vi "8532_V6.vi"(0 "enum":T11, 7 "set para":T10={"buffer size"=524288, "pci 8532 para"={"Ch"=[1, 1, 1, 1], "inputrange"=[1, 1, 1, 1], "采样频率"=10000, "耦合类型"=1, "预置触发计数器"=1024, "触发模式选择"=0, "ART通道选择"=0, "触发源"=0, "触发方向"=0, "当触发提前时，是否有效"=0, "时钟源"=0, "时钟输入输出源"=0, "是否将时钟信号输入到同步总线"=1}, "segment"={"nReadSizeWords"=8192, "nSegmentCount"=64, "nSegmentSizeWords"=8192}}, 11 "Main Vari in":T1={"Error"={"status"=FALSE, "code"=0, "source"=""}, "Test Info"={"Test Name"="", "Tester"=""}, "StateName"="", "Task Info"={"Accele Task"=[], "Simulate"=FALSE, "采样率"={"AISampleRate"=10123, "CouplingType"=10000, "Butter"=1000}, "Trig"={"PreTrigCNT"=0, "TriggerMode"=enum."中间触发", "TriggerSource"=enum."软件触发", "ATRTriggerChannel"=enum."通道0", "TriggerDir"=enum."下降沿触发", "TrigLevelVolt"=0.0, "bAvailableTrig"=FALSE}, "clock"={"EN"=FALSE, "clocksource"=enum."内部时钟", "outclocksource"=enum."Trig0"}, "delay(S)"=0.0}, "Virb Wave"=[{"t0"=timestamp(3350015091.8292503 s since 1904-01-01), "dt"=0.001, "Y"=array[1000 elements], "attributes"=variant("NI_ChannelName"=variant(string "PXI-6221/ai1"), "NI_UnitDescription"=variant(string "Deg C"))}], "Display Info"=[{"Frequency"=0.0, "RMS"=0.0}, {"Frequency"=0.0, "RMS"=0.0}, {"Frequency"=0.0, "RMS"=0.0}, {"Frequency"=0.0, "RMS"=0.0}, {"Frequency"=0.0, "RMS"=0.0}], "粉尘特性"={"名称"="", "粒径"="", "含水量"=""}, "测试条件"={"初始含氧量"="", "初始压力"="", "测试浓度"="", "点火能量"="", "初始温度"="", "反应器体积[L]"=0.0}, "ch size"=0} {"Task Info"."采样率"."CouplingType" items=["直流耦合", "交流耦合"]}) -> (3 "data?":bool, 6 "wave out":waveform(dbl)[](array[waveform]), 15 "Main Vari out":T1={"Error"={"status"=FALSE, "code"=0, "source"=""}, "Test Info"={"Test Name"="", "Tester"=""}, "StateName"="", "Task Info"={"Accele Task"=[], "Simulate"=FALSE, "采样率"={"AISampleRate"=10123, "CouplingType"=10000, "Butter"=1000}, "Trig"={"PreTrigCNT"=0, "TriggerMode"=enum."中间触发", "TriggerSource"=enum."软件触发", "ATRTriggerChannel"=enum."通道0", "TriggerDir"=enum."下降沿触发", "TrigLevelVolt"=0.0, "bAvailableTrig"=FALSE}, "clock"={"EN"=FALSE, "clocksource"=enum."内部时钟", "outclocksource"=enum."Trig0"}, "delay(S)"=0.0}, "Virb Wave"=[{"t0"=timestamp(3350015091.8292503 s since 1904-01-01), "dt"=0.001, "Y"=array[1000 elements], "attributes"=variant("NI_ChannelName"=variant(string "PXI-6221/ai1"), "NI_UnitDescription"=variant(string "Deg C"))}], "Display Info"=[{"Frequency"=0.0, "RMS"=0.0}, {"Frequency"=0.0, "RMS"=0.0}, {"Frequency"=0.0, "RMS"=0.0}, {"Frequency"=0.0, "RMS"=0.0}, {"Frequency"=0.0, "RMS"=0.0}], "粉尘特性"={"名称"="", "粒径"="", "含水量"=""}, "测试条件"={"初始含氧量"="", "初始压力"="", "测试浓度"="", "点火能量"="", "初始温度"="", "反应器体积[L]"=0.0}, "ch size"=0} {"Task Info"."采样率"."CouplingType" items=["直流耦合", "交流耦合"]})   [LabVIEW 2011]
uses:
  DAQ enum.ctl
  Ctrls/Sample Information.ctl
  Ctrls/Trig.ctl
  Ctrls/clock.ctl
  Ctrls/Task Info.ctl
  Ctrls/Main vari.ctl
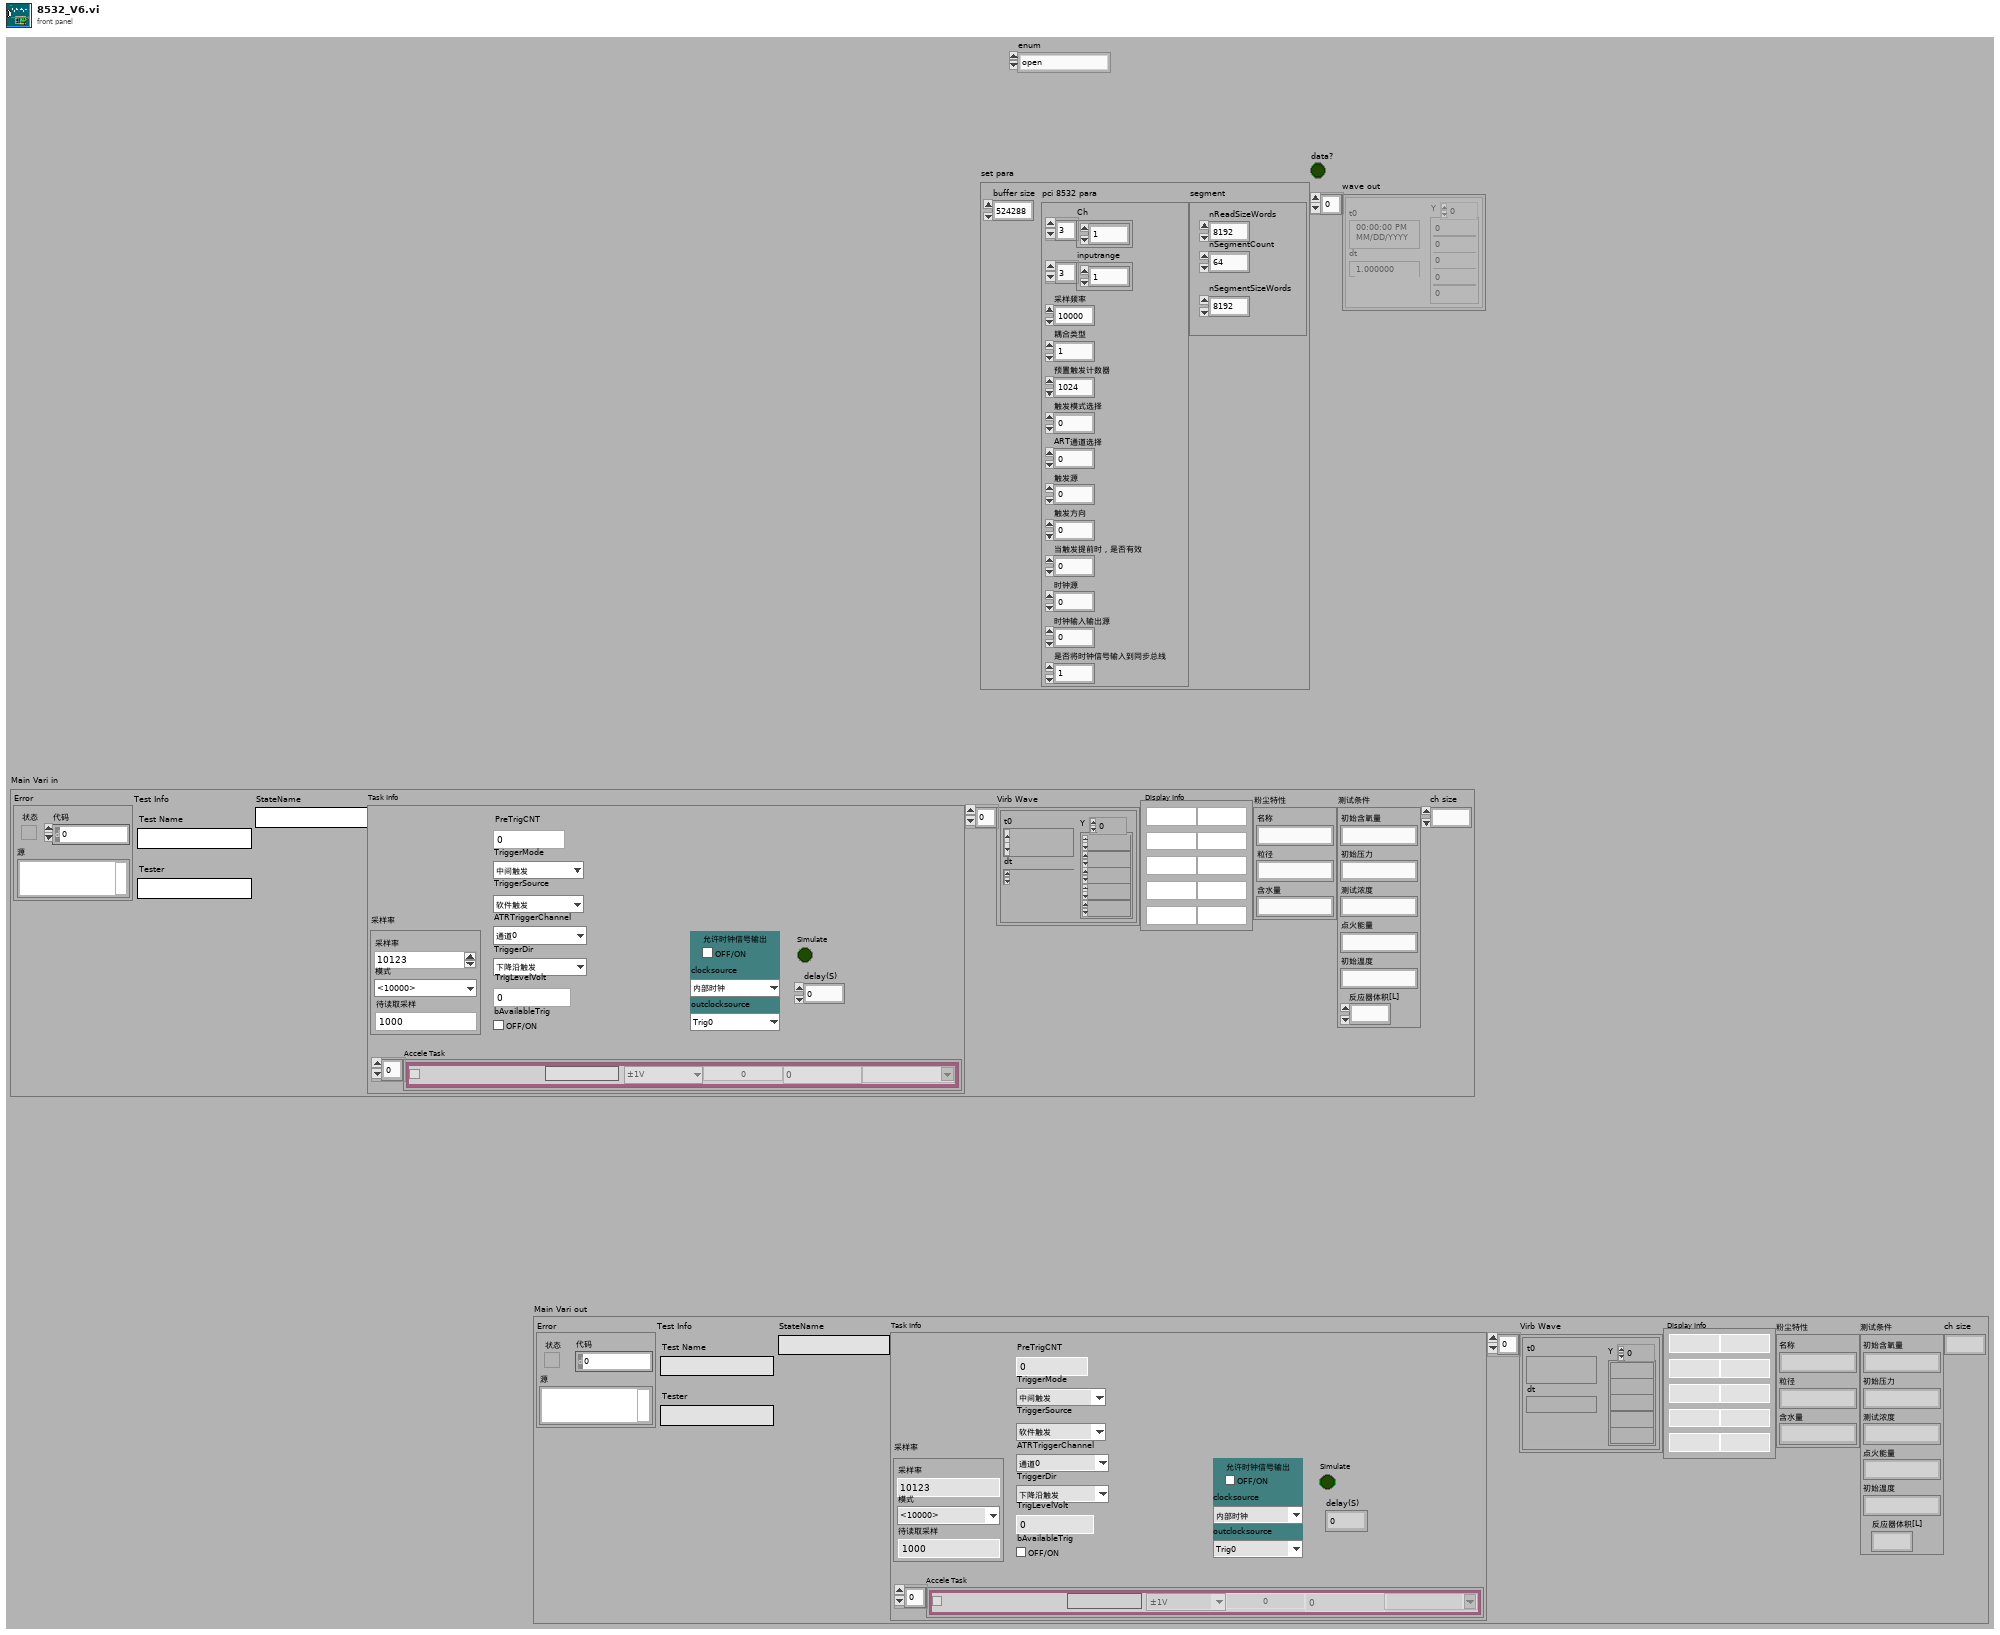
[diagram p1: front panel]
types:
  T1 = typedef "Main vari.ctl" = cluster{"Error":errorcluster, "Test Info":cluster{"Test Name":string, "Tester":string}, "StateName":string, "Task Info":T2, "Virb Wave":waveform(dbl)[], "Display Info":T7, "粉尘特性":T8, "测试条件":T9, "ch size":u8}
  T2 = typedef "Task Info.ctl" = cluster{"Accele Task":T3[], "Simulate":bool, "采样率":T4, "Trig":T5, "clock":T6, "delay(S)":dbl}
  T3 = typedef "Acceleration Channel Config_Ctrls-某型振动实验台测试系统.ctl" = cluster{"Enable":bool, "Name":string, "range":enum16{"±1V", "±5V"}, "SensValue":dbl, "PhysicalName":string, "off":dbl, "Sensunits":string}
  T4 = typedef "Sample Information.ctl" = cluster{"AISampleRate":i32, "CouplingType":i32, "Butter":i32}
  T5 = typedef "Trig.ctl" = cluster{"PreTrigCNT":i32, "TriggerMode":enum16{"中间触发", "后触发", "预触发", "硬件延时触发"}, "TriggerSource":enum16{"软件触发", "DTR信号源", "ATR信号源", "Triger信号触发"}, "ATRTriggerChannel":enum16{"通道0", "通道1", "通道2", "通道3"}, "TriggerDir":enum16{"下降沿触发", "上升沿触发", "上下边没均触发"}, "TrigLevelVolt":sgl, "bAvailableTrig":bool}
  T6 = typedef "clock.ctl" = cluster{"EN":bool, "clocksource":enum16{"内部时钟", "外部时钟"}, "outclocksource":enum16{"Trig0", "Trig1", "Trig2", "Trig3", "Trig4", "Trig5", "Trig6", "Trig7", "PXI_STAR"}}
  T7 = typedef "Display Information_Ctrls-某型振动实验台测试系统.ctl" = cluster{"Frequency":dbl, "RMS":dbl}[]
  T8 = typedef "粉尘特性.ctl" = cluster{"名称":string, "粒径":string, "含水量":string}
  T9 = typedef "测试条件.ctl" = cluster{"初始含氧量":string, "初始压力":string, "测试浓度":string, "点火能量":string, "初始温度":string, "反应器体积[L]":dbl}
  T10 = cluster{"buffer size":i32, "pci 8532 para":cluster{"Ch":i32[], "inputrange":i32[], "采样频率":i32, "耦合类型":i32, "预置触发计数器":i32, "触发模式选择":i32, "ART通道选择":i32, "触发源":i32, "触发方向":i32, "当触发提前时，是否有效":i32, "时钟源":i32, "时钟输入输出源":i32, "是否将时钟信号输入到同步总线":i32}, "segment":cluster{"nReadSizeWords":i32, "nSegmentCount":i32, "nSegmentSizeWords":i32}}
  T11 = typedef "DAQ enum.ctl" = enum16{"open", "config", "start", "read", "stop", "noop", "close"}
  T12 = cluster{"Device":i32, "Event":i32, "state":i32[]}
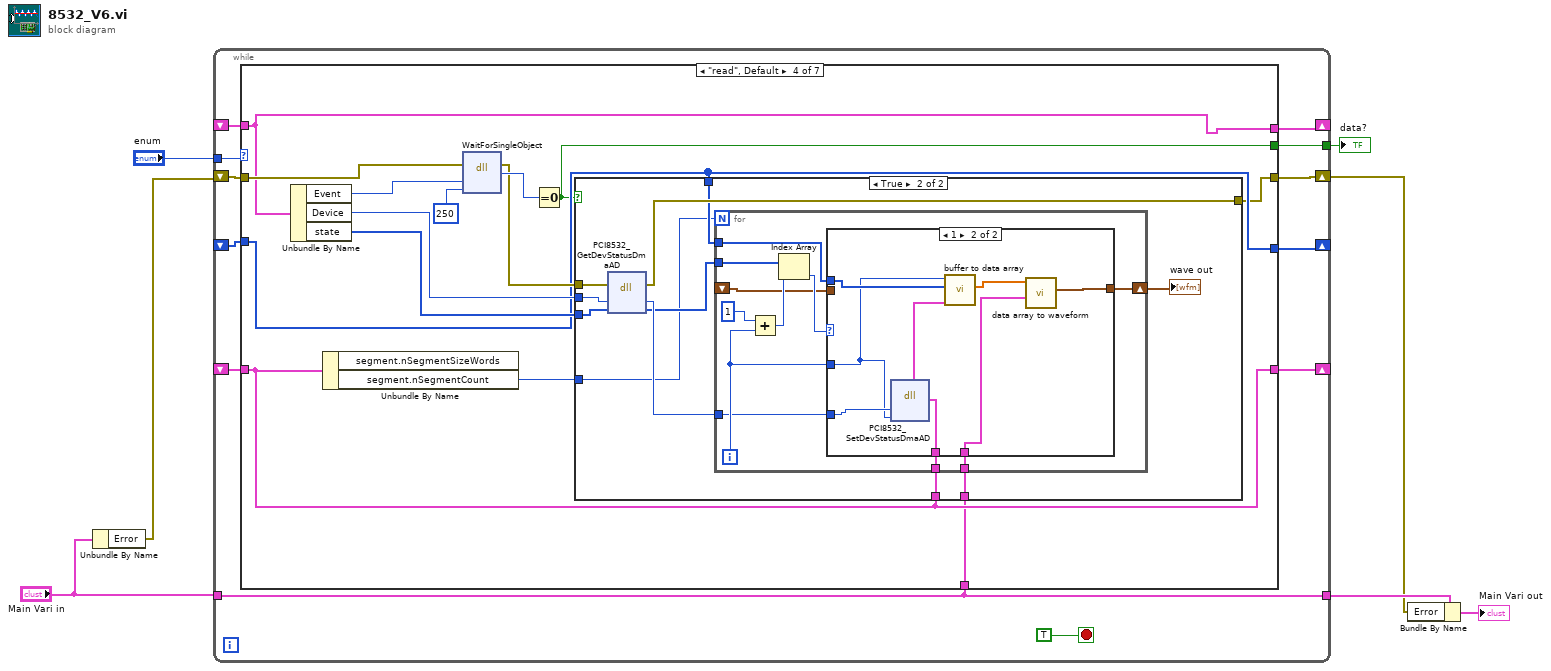
[diagram p0: block diagram]
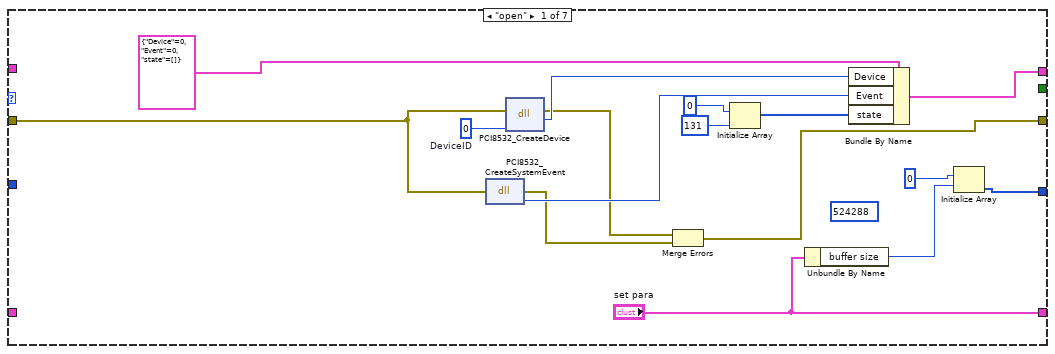
[diagram p2: hidden frame]
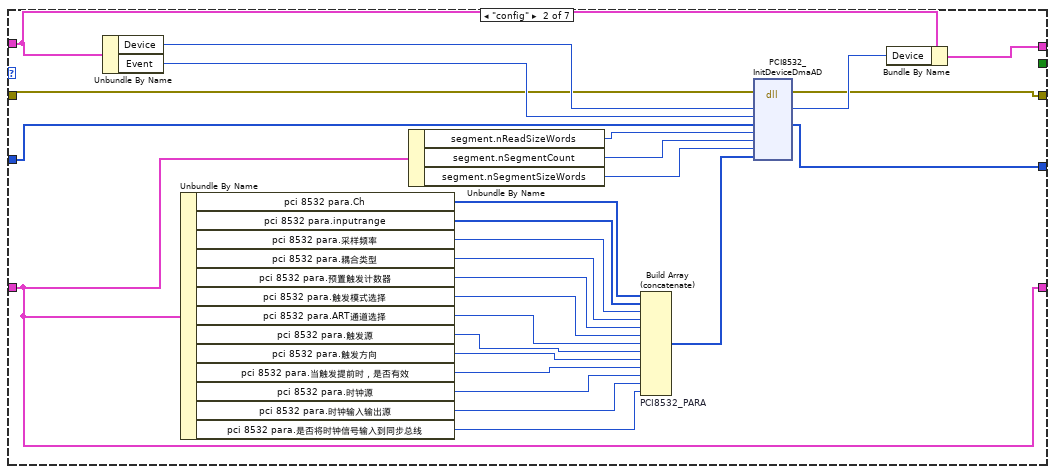
[diagram p3: hidden frame]
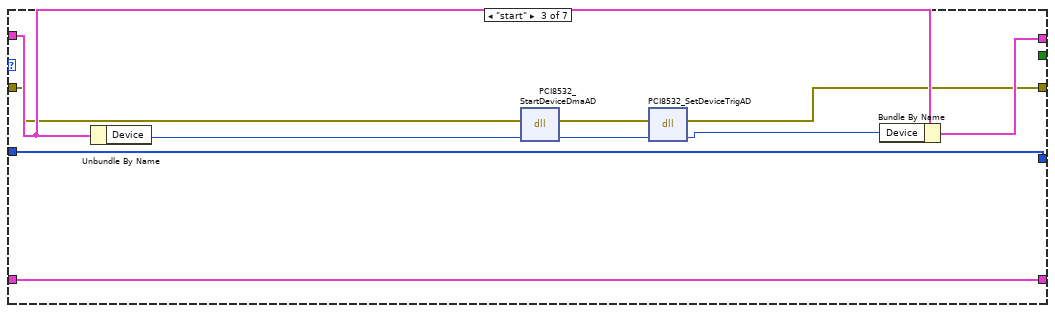
[diagram p4: hidden frame]
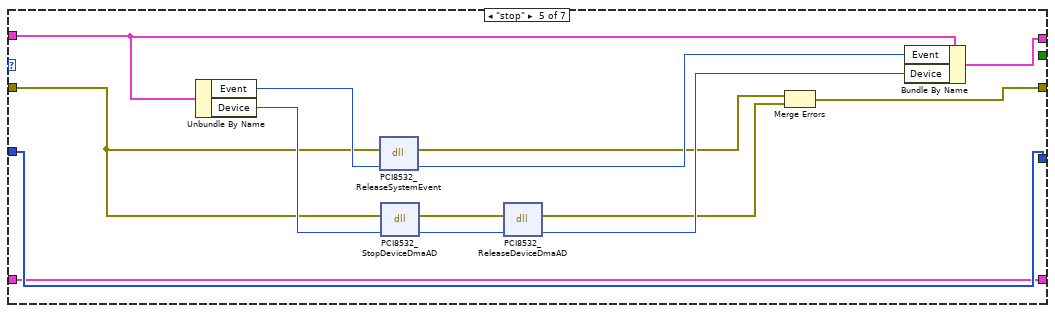
[diagram p7: hidden frame]
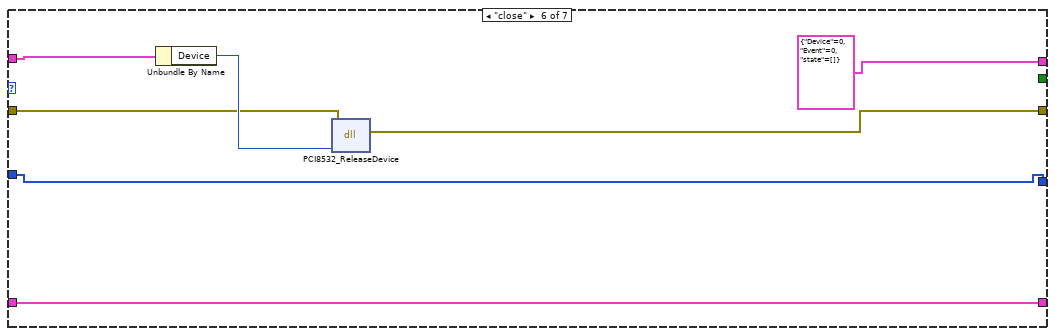
[diagram p8: hidden frame]
diagram:
  n1 = Unbundle By Name("Main Vari in") -> ("Error"=w4:errorcluster)
  n2 = while {
    tunnel: "enum" -> [w18]
    shift-right: [w16] -> _
    shift-left: _ -> [w17]
    shift-right: [w15] -> _
    shift-left: _ -> [w14]
    shift-right: [w12] -> w1
    shift-left: w4 -> [w13]
    shift-right: [w11] -> _
    shift-left: _ -> [w10]
    tunnel: [w9] -> w6
    tunnel: "Main Vari in" -> [w8]
    tunnel: [w8] -> w3
    stop <- TRUE stop-if-true
    n3 = case shown="\"read\", Default" w18 {
      tunnel: w17 -> [_ w58 w68 w78 w129 w138 w142]
      tunnel: [w34 w59 w69 w78 w128 T12 {"Device"=0, "Event"=0, "state"=[]} ("var in") w142] -> w16
      tunnel: [w25 w36 w66 w80 w121 w136 w141] -> w15
      tunnel: w14 -> [_ w56 w66 w80 w121 w136 w141]
      tunnel: w13 -> [w23 w54 w64 w79 w120 w133 w140]
      tunnel: [w22 w55 w65 w77 w119 w134 w140] -> w12
      tunnel: ["set para" w37 w63 w74 w118 w132 w139] -> w11
      tunnel: w10 -> [_ w37 w63 w74 w118 w132 w139]
      tunnel: [_ _ _ w76 _ _ _] -> w9
      tunnel: w8 -> [_ _ _ w73 _ _ _]
      frame "open" {
        (unwired) 524288 ("dimension size")
        w35 = 0  # DeviceID
        n4 = dll-call lib="PCI8532_32" fn="PCI8532_CreateSystemEvent" ("CreateSystemEvent")(error in=w23) -> (error out=w26:errorcluster, "hEvent"=w32:i32)  [unwired: 2 in, 1 out]
        n5 = dll-call lib="PCI8532_32" fn="PCI8532_CreateDevice" label="CreateDevice"(error in=w23, "DeviceID"=w35) -> (error out=w27:errorcluster, w33:i32)  [unwired: 3 in, 1 out]
        n6 = Merge Errors(w27, w26) -> (w22:errorcluster)
        n7 = Initialize Array(0 ("element"), 131 ("dimension size")) -> (w28:i32[])
        n8 = Unbundle By Name("set para") -> ("buffer size"=w20:i32)
        n9 = Bundle By Name(cluster=T12 {"Device"=0, "Event"=0, "state"=[]} ("var in"), "Device"=w33, "Event"=w32, "state"=w28) -> (w34:T12)
        n10 = Initialize Array(u16 0, w20) -> (w25:u16[])
      }
      frame "config" {
        n11 = Unbundle By Name(w58) -> ("Device"=w61:i32, "Event"=w60:i32)
        n12 = Unbundle By Name(w37) -> ("pci 8532 para.Ch"=w50:i32[], "pci 8532 para.inputrange"=w49:i32[], "pci 8532 para.采样频率"=w48:i32, "pci 8532 para.耦合类型"=w47:i32, "pci 8532 para.预置触发计数器"=w46:i32, "pci 8532 para.触发模式选择"=w45:i32, "pci 8532 para.ART通道选择"=w44:i32, "pci 8532 para.触发源"=w43:i32, "pci 8532 para.触发方向"=w42:i32, "pci 8532 para.当触发提前时，是否有效"=w41:i32, "pci 8532 para.时钟源"=w40:i32, "pci 8532 para.时钟输入输出源"=w39:i32, "pci 8532 para.是否将时钟信号输入到同步总线"=w38:i32)
        n13 = Unbundle By Name(w37) -> ("segment.nReadSizeWords"=w53:i32, "segment.nSegmentCount"=w52:i32, "segment.nSegmentSizeWords"=w51:i32)
        n14 = Build Array (concatenate) "PCI8532_PARA"(w50, w49, w48, w47, w46, w45, w44, w43, w42, w41, w40, w39, w38) -> (w62:i32[])
        n15 = dll-call lib="PCI8532_32" fn="PCI8532_InitDeviceDmaAD" label="InitDeviceDmaAD"(error in=w54, "hDevice"=w61, "hDmaEvent"=w60, "ADBuffer"=w56, "nReadSizeWords"=w53, "nSegmentCount"=w52, "nSegmentSizeWords"=w51, "pAPara"=w62) -> (error out=w55:errorcluster, "hDevice"=w57:i32, "ADBuffer"=w36:u16[])  [unwired: 8 in, 1 out]
        n16 = Bundle By Name(cluster=w58, "Device"=w57) -> (w59:T12)
      }
      frame "start" {
        n17 = Unbundle By Name(w68) -> ("Device"=w70:i32)
        n18 = dll-call lib="PCI8532_32" fn="PCI8532_StartDeviceDmaAD" label="StartDeviceDmaAD"(error in=w64, "hDevice"=w70) -> (error out=w71:errorcluster, "hDevice"=w72:i32)  [unwired: 3 in, 1 out]
        n19 = dll-call lib="PCI8532_32" fn="PCI8532_SetDeviceTrigAD" label="SetDeviceTrigAD"(error in=w71, "hDevice"=w72) -> (error out=w65:errorcluster, "hDevice"=w67:i32)  [unwired: 3 in, 1 out]
        n20 = Bundle By Name(cluster=w68, "Device"=w67) -> (w69:T12)
      }
      frame "read", Default {
        n21 = Unbundle By Name(w78) -> ("Event"=w85:i32, "Device"=w82:i32, "state"=w81:i32[])
        n22 = Unbundle By Name(w74) -> ("segment.nSegmentCount"=w75:i32)  [unwired: 1 out]
        n23 = dll-call lib="kernel32" fn="WaitForSingleObject"(error in=w79, "hEvent"=w85, "dwMilliseconds"=250 ("millisecond multiple")) -> (error out=w83:errorcluster, w84:u32)  [unwired: 4 in, 1 out]
        n24 = Equal To 0?(x=w84) -> (x = 0?=w76:bool)
        n25 = case shown="True" w76 {
          tunnel: w83 -> [w87 w98]
          tunnel: [w87 w97] -> w77
          tunnel: w82 -> [_ w96]
          tunnel: w81 -> [_ w95]
          tunnel: w80 -> [_ w93]
          tunnel: w75 -> [_ w91]
          tunnel: w74 -> [_ w90]
          tunnel: w73 -> [_ w88]
          frame False {
          }
          frame True {
            n26 = dll-call lib="PCI8532_32" fn="PCI8532_GetDevStatusDmaAD" ("GetDevStatusDmaAD")(error in=w98, "hDevice"=w96, "pDMAStatus"=w95) -> (error out=w97:errorcluster, "hDevice"=w94:i32, "pDMAStatus"=w92:i32[])  [unwired: 3 in, 1 out]
            n27 = for {
              N: w91 -> [_]
              tunnel: w92 -> [w109]
              tunnel: w93 -> [w107]
              tunnel: w94 -> [w103]
              tunnel: w90 -> [w102]
              shift-right: [w101] -> w89
              shift-left: _ -> [w100]
              tunnel: w88 -> [w99]
              i -> [w105]
              n28 = Add(x=1, y=w105) -> (x+y=w104:i32)
              n29 = Index Array(array=w109, index=w104) -> (element=w108:i32)
              n30 = case shown="1" w108 {
                tunnel: w105 -> [_ w115]
                tunnel: w107 -> [_ w116]
                tunnel: w103 -> [_ w117]
                tunnel: w102 -> [_ w112]
                tunnel: [w110 w114] -> w101
                tunnel: w100 -> [w110 _]
                tunnel: w99 -> [_ w111]
                frame 0, Default {
                }
                frame 1 {
                  n31 = dll-call lib="PCI8532_32" fn="PCI8532_SetDevStatusDmaAD" ("SetDevStatusDmaAD")("hDevice"=w117, "iClrBufferID"=w115) -> ()  [unwired: 6 in, 2 out]
                  n32 = call "buffer to data array.vi"("set para 2"=w112, "buffer"=w116, "i"=w115) -> ("data"=w113:dbl[])  [unwired: 2 in, 6 out]
                  n33 = call "data array to waveform.vi"("Main Vari"=w111, "data"=w113) -> ("wave out"=w114:waveform(dbl)[])  [unwired: 2 in, 7 out]
                }
              }
            }
            "wave out" <- w89
          }
        }
      }
      frame "stop" {
        n34 = Unbundle By Name(w129) -> ("Event"=w130:i32, "Device"=w122:i32)
        n35 = dll-call lib="PCI8532_32" fn="PCI8532_ReleaseSystemEvent" label="ReleaseSystemEvent"(error in=w120, "hEvent"=w130) -> (error out=w125:errorcluster, "hEvent"=w127:i32)  [unwired: 3 in, 1 out]
        n36 = dll-call lib="PCI8532_32" fn="PCI8532_StopDeviceDmaAD" label="StopDeviceDmaAD"(error in=w120, "hDevice"=w122) -> (error out=w123:errorcluster, "hDevice"=w131:i32)  [unwired: 3 in, 1 out]
        n37 = dll-call lib="PCI8532_32" fn="PCI8532_ReleaseDeviceDmaAD" label="ReleaseDeviceDmaAD"(error in=w123, "hDevice"=w131) -> (error out=w124:errorcluster, "hDevice"=w126:i32)  [unwired: 3 in, 1 out]
        n38 = Merge Errors(w125, w124) -> (w119:errorcluster)
        n39 = Bundle By Name(cluster=w129, "Event"=w127, "Device"=w126) -> (w128:T12)
      }
      frame "close" {
        n40 = Unbundle By Name(w138) -> ("Device"=w137:i32)
        n41 = dll-call lib="PCI8532_32" fn="PCI8532_ReleaseDevice" label="ReleaseDevice"(error in=w133, "hDevice"=w137) -> (error out=w134:errorcluster)  [unwired: 4 in, 1 out]
      }
      frame "noop" {
      }
    }
  }
  "data?" <- w6
  n42 = Bundle By Name(cluster=w3, "Error"=w1) -> (→"Main Vari out":T1)
